vi "peakFinding remBL2.vi"(11 "smoothData":cluster{"xData":dbl[], "yData":dbl[]}) -> (3 "peakData":cluster{"xData":dbl[], "newYData":dbl[]})   [LabVIEW 2018]
panel:
  in  "itermax":i32
  in  "lambda":i32=100
  out "noBaseline":cluster{"xData":dbl[], "yData":dbl[]}(graph)
  out "calcProcess":cluster{"xData":dbl[], "yData":dbl[]}(graph)
  out "rawData":cluster{"xData":dbl[], "yData":dbl[]}(graph)
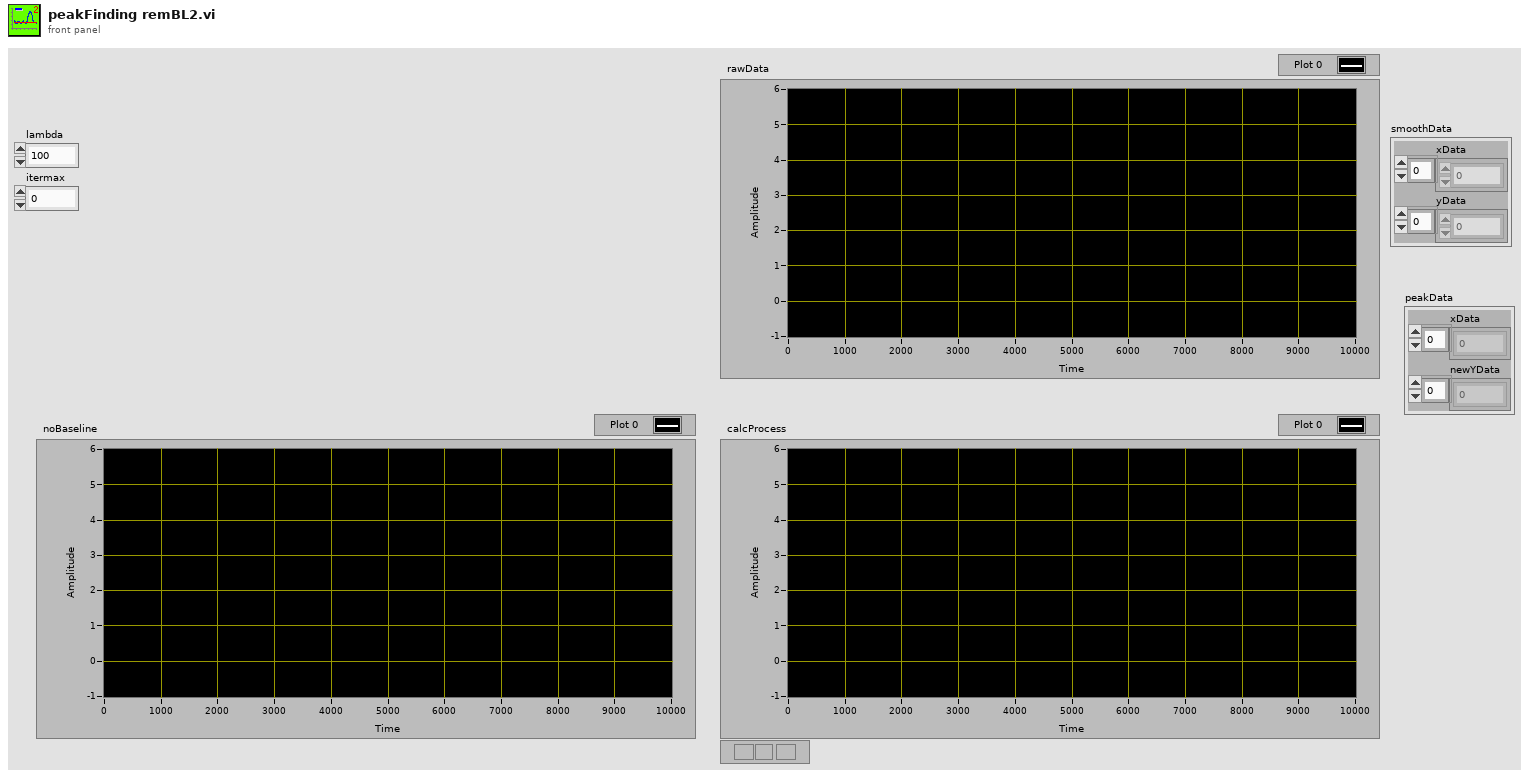
[diagram p1: front panel]
types:
  T1 = typedef "NI_Matrix.lvlib/RealMatrix.ctl" = dbl[][]
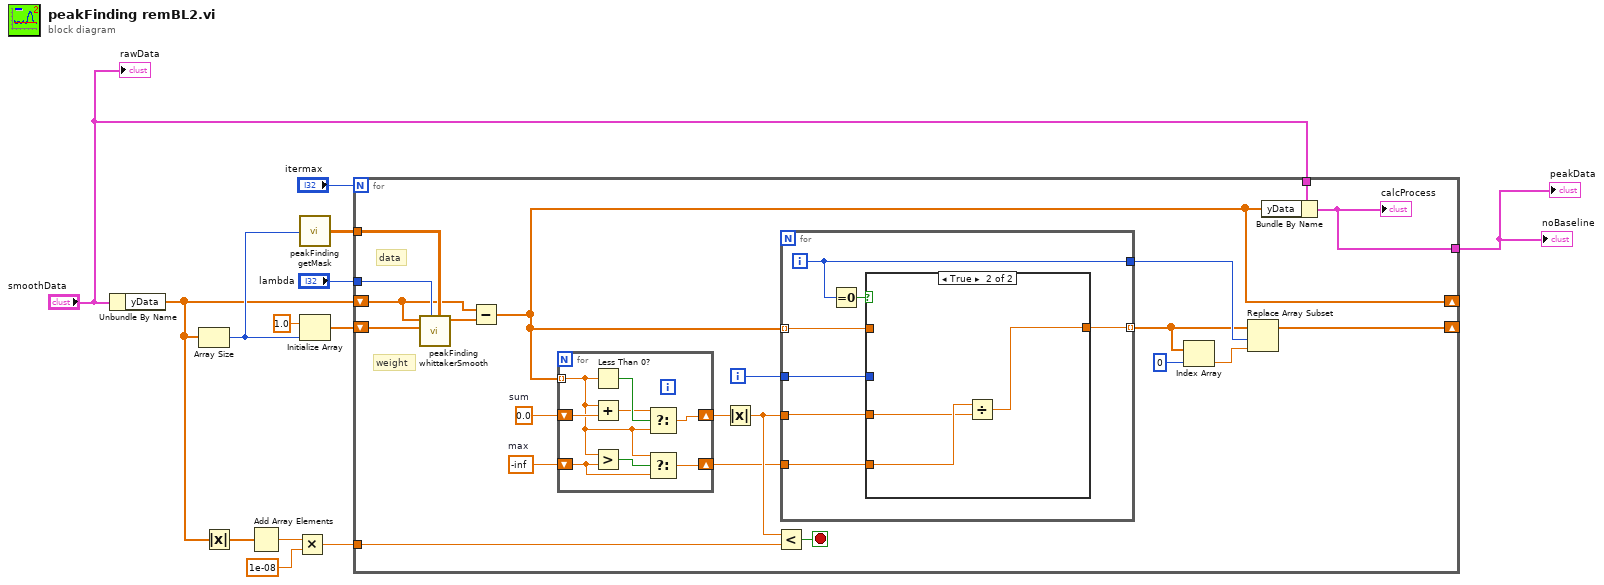
[diagram p0: block diagram]
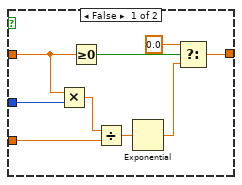
[diagram p2: hidden frame]
diagram:
  n1 = Unbundle By Name("smoothData") -> ("yData"=w3:dbl[])
  n2 = Array Size(array=w3) -> (size(s)=w11:i32)
  n3 = Absolute Value(x=w3) -> (abs(x)=w8:dbl[])
  n4 = Add Array Elements(numeric array=w8) -> (sum=w7:dbl)
  n5 = Multiply(x=w7, y=1e-08) -> (x*y=w5:dbl)
  n6 = call "peakFinding getMask.vi"("dataArraySize"=w11) -> ("diffMatrix"=w10:T1)
  n7 = Initialize Array(1.0 ("element"), w11) -> (w12:dbl[])
  n8 = for {
    N: "itermax" -> [_]
    tunnel: w10 -> [w33]
    tunnel: "lambda" -> [w32]
    shift-right: [w18] -> _
    shift-left: w12 -> [w34]
    tunnel: w5 -> [w26]
    tunnel: "smoothData" -> [w16]
    tunnel: [w15] -> w1
    shift-right: [w14] -> _
    shift-left: w3 -> [w17]
    i -> [w25]
    stop <- w27 stop-if-true
    w29 = -inf  # max
    w30 = 0.0  # sum
    # "data"
    # "weight"
    n9 = call "peakFinding whittakerSmooth.vi"("diffMatrix"=w33, "lambda"=w32, "weight"=w34, "data"=w17) -> ("background"=w31:dbl[])  [unwired: 7 in]
    n10 = Subtract(x=w17, y=w31) -> (x-y=w14:dbl[])
    n11 = for {
      tunnel: w14 -> [w56] mode=indexing
      shift-right: [w58] -> w28
      shift-left: w30 -> [w60]
      shift-right: [w54] -> w23
      shift-left: w29 -> [w55]
      n12 = Less Than 0?(x=w56) -> (x < 0?=w61:bool)
      n13 = Add(x=w56, y=w60) -> (x+y=w59:dbl)
      n14 = Greater?(x=w56, y=w55) -> (0:w57:bool)
      n15 = Select(t=w59, s=w61, f=w56) -> (s? t:f=w58:dbl)
      n16 = Select(t=w56, s=w57, f=w55) -> (s? t:f=w54:dbl)
    }
    n17 = Absolute Value(x=w28) -> (abs(x)=w24:dbl)
    n18 = Less?(x=w24, y=w26) -> (x < y?=w27:bool)
    n19 = for {
      tunnel: w14 -> [w39] mode=indexing
      tunnel: [w41] -> w19 mode=indexing
      tunnel: w25 -> [w38]
      tunnel: w24 -> [w40]
      tunnel: [w37] -> w20
      tunnel: w23 -> [w35]
      i -> [w37]
      n20 = Equal To 0?(x=w37) -> (x = 0?=w36:bool)
      n21 = case shown="True" w36 {
        tunnel: [w48 w51] -> w41
        tunnel: w40 -> [w47 w52]
        tunnel: w39 -> [w46 _]
        tunnel: w38 -> [w45 _]
        tunnel: w35 -> [_ w53]
        frame False {
          n22 = Multiply(x=w46, y=w45) -> (x*y=w44:dbl)
          n23 = Greater Or Equal To 0?(x=w46) -> (x >= 0?=w50:bool)
          n24 = Divide(x=w44, y=w47) -> (x/y=w43:dbl)
          n25 = Exponential(1:w43) -> (0:w42:dbl)
          n26 = Select(t=0.0, s=w50, f=w42) -> (s? t:f=w48:dbl)
        }
        frame True {
          n27 = Divide(x=w53, y=w52) -> (x/y=w51:dbl)
        }
      }
    }
    n28 = Index Array(array=w19, index=0) -> (element=w21:dbl)
    n29 = Replace Array Subset(array=w19, new element=w21, index=w20) -> (w18:dbl[])
    n30 = Bundle By Name(cluster=w16, "yData"=w14) -> (w15:cluster{"xData":dbl[], "yData":dbl[]})
    "calcProcess" <- w15
  }
  "peakData" <- w1
  "noBaseline" <- w1
  "rawData" <- "smoothData"
